vi "Load Plugin Front Panel.vi"(8 "error in (no error)":errorcluster, 10 "Sub Panel":refnum<vi>, 11 "Generic Controller in":refnum<class "Generic Plugin.lvclass">) -> (0 "error out":errorcluster)   [LabVIEW 2020, in "RxnRover.lvlib"]
uses:
  RxnRover.lvlib
  Plugin Servers/Controller/Generic Plugin.lvclass
  Plugin Servers/Controller/Generic Plugin.lvclass/Generic Plugin.ctl
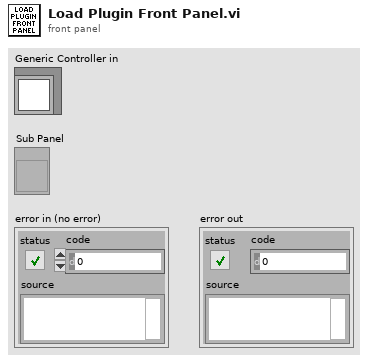
[diagram p1: front panel]
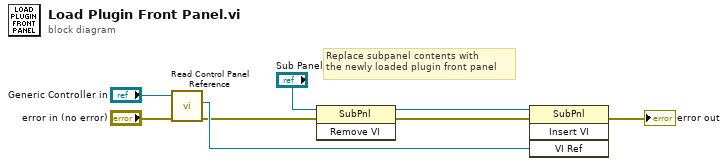
[diagram p0: block diagram]
diagram:
  # "Replace subpanel contents with \nthe newly loaded plugin front panel"
  n1 = call "Read Control Panel Reference.vi"("error in (no error)"="error in (no error)", "controller in"="Generic Controller in") -> ("error out"=w2:errorcluster, "Control Panel Reference"=w6:refnum<vi>)  [unwired: 7 in, 1 out]
  n2 = invoke on="Invoke Node" class="SubPnl" method="Remove VI"(reference="Sub Panel", error in=w2) -> (reference out=w7:refnum<vi>, error out=w1:errorcluster)  [unwired: 1 in, 1 out]
  n3 = invoke on="Invoke Node" class="SubPnl" method="Insert VI"(reference=w7, error in=w1, "VI Ref"=w6) -> (error out=→"error out":errorcluster)  [unwired: 1 in, 3 out]
